vi "Bronkhorst FLOW-BUS Setpoint Configure and Read.vi"() -> ()   [LabVIEW 2021]
doc: "This VI sets the Setpoint Percentage value in the instrument. Then the Setpoint Direct value, and the Capacity Unit are read from the instrument. To use this VI, select the node address and the correct COM port before running the example."
uses:
  <instrlib>/Bronkhorst FLOW-BUS/Public/Configure/Setpoint/Configure Setpoint (Percentage).vi
  <instrlib>/Bronkhorst FLOW-BUS/Public/Data/Setpoint/Read Setpoint (Direct).vi
  <instrlib>/Bronkhorst FLOW-BUS/Bronkhorst FLOW-BUS.lvlib
panel:
  in  "Baud Rate (38400)":u32(ring)=38400 items=["9600"=9600, "19200"=19200, "38400"=38400, "57600"=57600, "115200"=115200, "230400"=230400, "460800"=460800]
  out "Capacity Unit":string
  out "Setpoint Direct":sgl
  in  "Setpoint Percentage (0%)":dbl min=0.0 max=100.0 step=1.0 format="%#.2g"
  in  "Node (3)":u8=3 caption="Node" min=3 max=128 step=1
  in  "VISA resource name":refnum<visa-resource-name>
  # "(c) 2014 Bronkhorst High-Tech B.V.  ALL RIGHTS RESERVED."
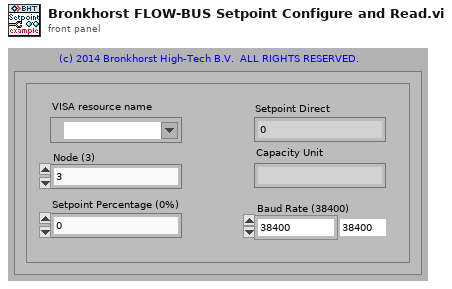
[diagram p1: front panel]
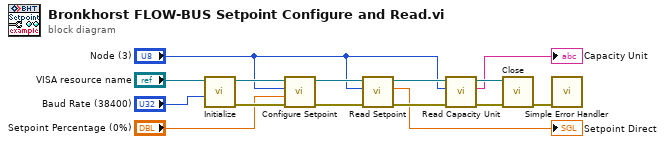
[diagram p0: block diagram]
diagram:
  n1 = call <instrlib>:"Initialize.vi"("Baud Rate (38400)"="Baud Rate (38400)", "VISA resource name"="VISA resource name") -> ("error out"=w11:errorcluster, "VISA resource name out"=w10:refnum<visa-resource-name>)  [unwired: 8 in]
  n2 = call-poly <instrlib>:"Configure Setpoint.vi"("error in (no error)"=w11, "Setpoint Percentage (0%)"="Setpoint Percentage (0%)", "Node (3)"="Node (3)", "VISA resource name"=w10) -> ("error out"=w6:errorcluster, "VISA resource name out"=w5:refnum<visa-resource-name>)  [unwired: 6 in]
  n3 = call-poly <instrlib>:"Read Setpoint.vi"("error in (no error)"=w6, "Node (3)"="Node (3)", "VISA resource name"=w5) -> ("error out"=w8:errorcluster, "Setpoint Direct"=→"Setpoint Direct":sgl, "VISA resource name out"=w9:refnum<visa-resource-name>)  [unwired: 6 in]
  n4 = call <instrlib>:"Read Capacity Unit.vi"("error in (no error)"=w8, "Node (3)"="Node (3)", "VISA resource name"=w9) -> ("error out"=w14:errorcluster, "Capacity Unit"=→"Capacity Unit":string, "VISA resource name out"=w13:refnum<visa-resource-name>)  [unwired: 6 in]
  n5 = call <instrlib>:"Close.vi"("error in (no error)"=w14, "VISA resource name"=w13) -> ("error out"=w1:errorcluster)  [unwired: 9 in]
  n6 = call <vilib>:"Simple Error Handler.vi"("error in (no error)"=w1) -> ()  [unwired: 4 in, 5 out]
